vi "puff_stimulus_advanced.vi"(2 "Input Array":dbl[](array[numeric]), 3 "Cluster":T1) -> (0 "Timing array changed?":bool, 1 "Output Array":dbl[](array[numeric]))   [LabVIEW 2015]
panel:
  in  "Puff Stimulus Duration(ms)":i32[][](array[numeric]) min=4 max=65535
  in  "Fraction of time between is active":sgl[][](array[numeric]) min=5e-06 max=0.99995
  in  "stop":bool
  in  "OK Button":bool
  in  "Puff Stimulus Timing Array":dbl[](array[numeric])
  # "Duty Cycle"
  # "Switch time (ms)"
  # "Puff Stimulus Timing Array (ms)"
  # "Trigger signal duration (ms)"
  # "Switch time (ms)"
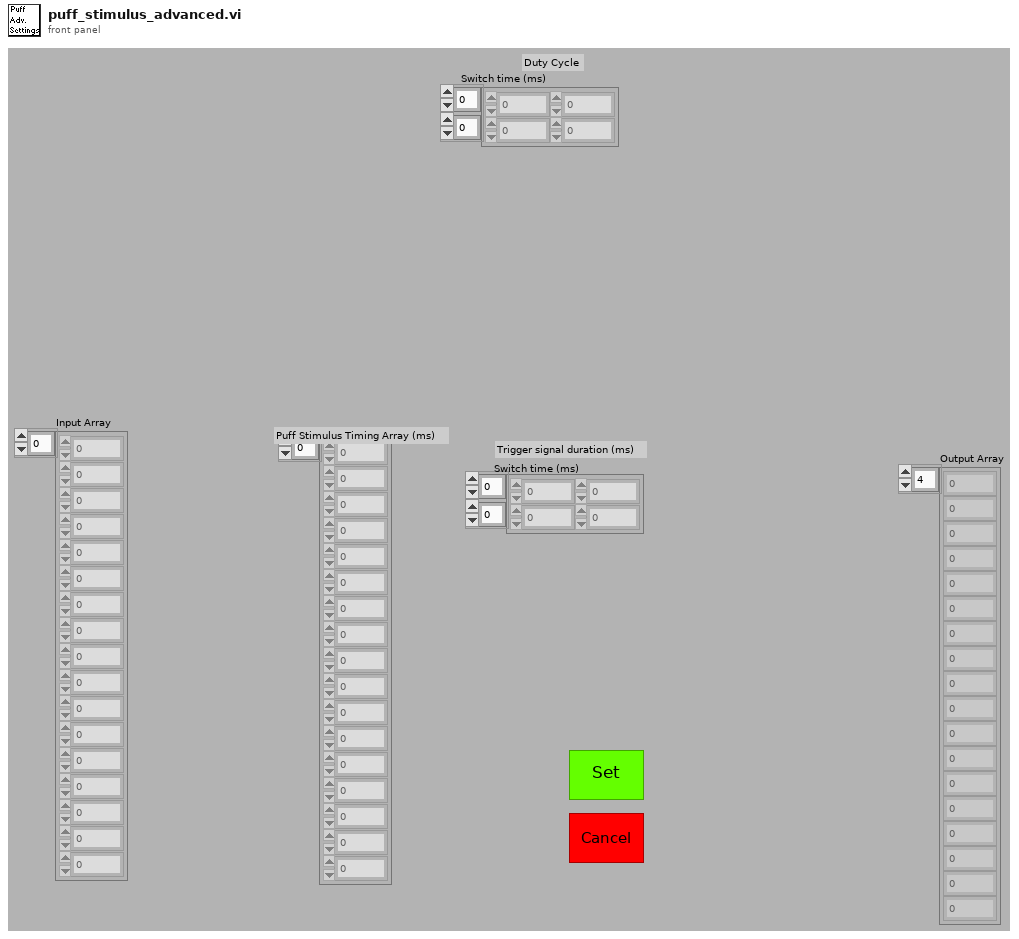
[diagram p1: front panel]
types:
  T1 = cluster{"puff fraction of time between is active":refnum<vi>, "time between puff onset":refnum<vi>}
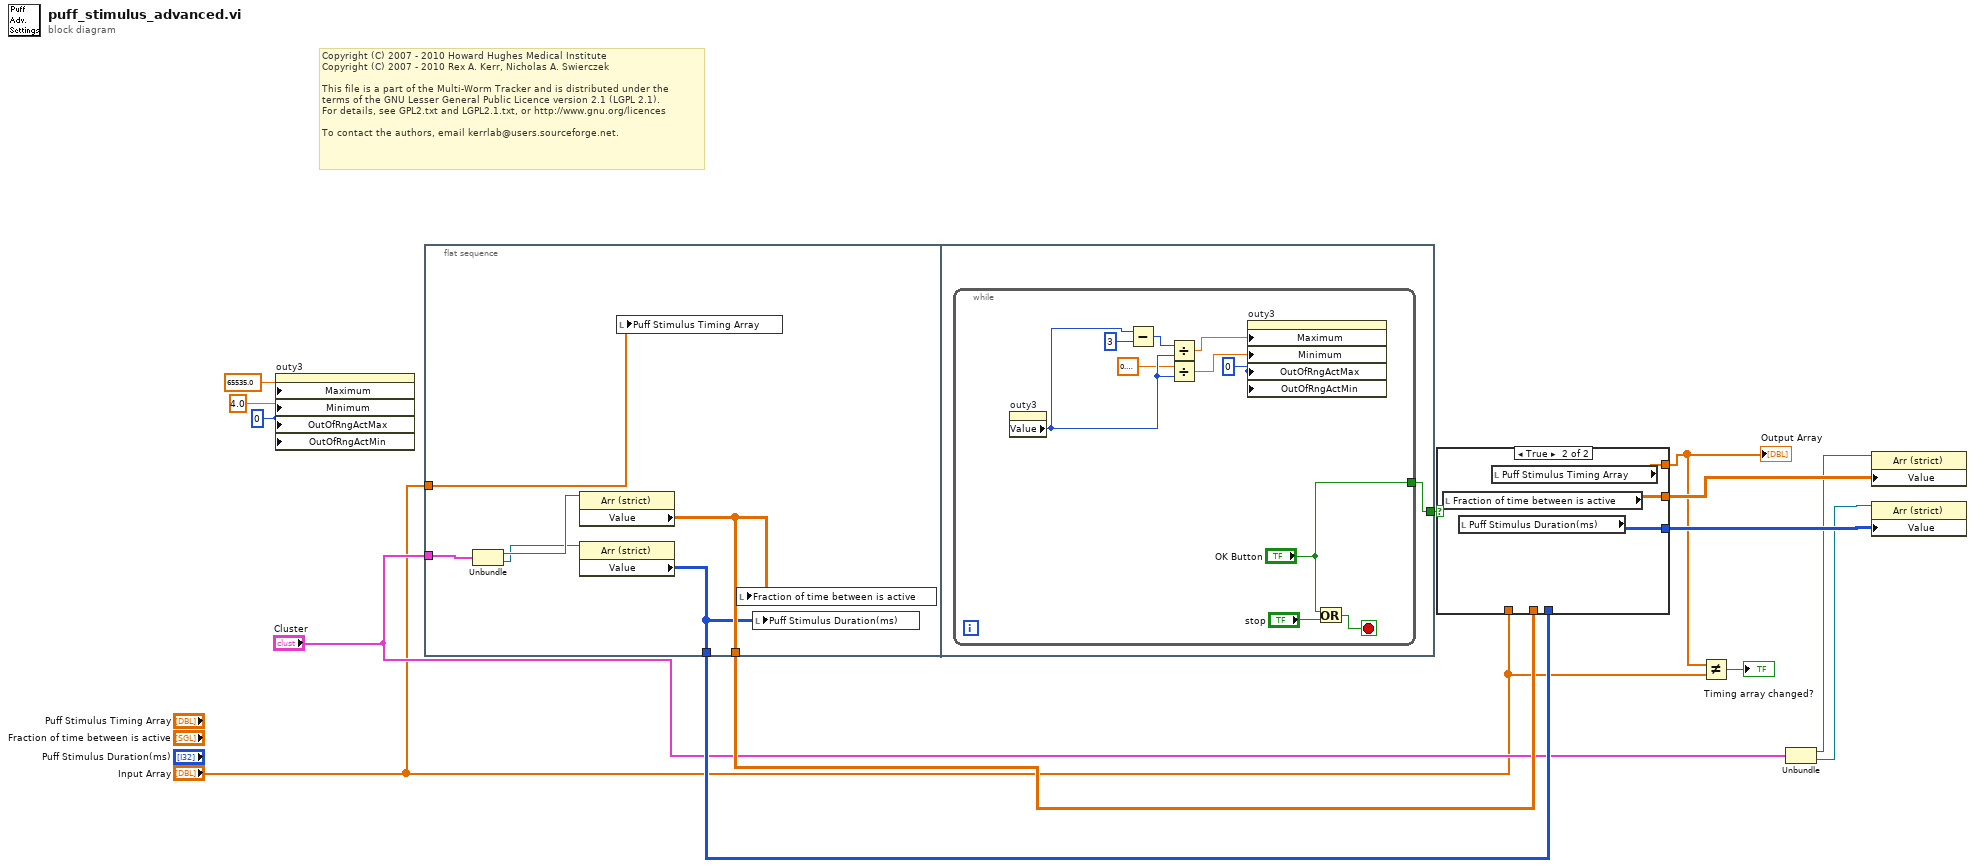
[diagram p0: block diagram]
diagram:
  w7 = u8 0 ("Response to Value Outside Limits:Maximum")
  # "Copyright (C) 2007 - 2010 Howard Hughes Medical Institute\nCopyright (C) 2007 - 2010 Rex A. Kerr, Nicholas A. Swierczek\n \nThis file is a part of the Multi-Worm Tracker and is distributed under the\nterms of the GNU Lesser General Public Licence version 2.1 (LGPL 2.1).\nFor details, see GPL2.txt and LGPL2.1.txt, or http://www.gnu.org/licences\n \nTo contact the authors, email kerrlab@users.sourceforge.net."
  n1 = property on="outy3" class="DigNum (strict)"("Maximum"=65535.0 ("x"), "Minimum"=4.0 ("Data Entry Limits:Minimum"), "OutOfRngActMax"=w7, "OutOfRngActMin"=w7) -> ()  [unwired: 2 in, 2 out]
  n2 = flat-sequence {
    tunnel: "Input Array" -> [w20]
    tunnel: "Cluster" -> [w19]
    tunnel: [w18] -> w6
    tunnel: [w17] -> w5
    tunnel: [w21] -> w14
    frame #0 {
      n3 = Unbundle(w19) -> ("puff fraction of time between is active"=w16:refnum<vi>, "time between puff onset"=w15:refnum<vi>)
      n4 = property class="Arr (strict)"(reference=w16) -> ("Value"=w18:sgl[][])  [unwired: 1 in, 2 out]
      n5 = property class="Arr (strict)"(reference=w15) -> ("Value"=w17:i32[][])  [unwired: 1 in, 2 out]
      n6 = local write "Puff Stimulus Timing Array"(w20) -> ()
      n7 = local write "Fraction of time between is active"(w18) -> ()
      n8 = local write "Puff Stimulus Duration(ms)"(w17) -> ()
    }
    frame #1 {
      n9 = while {
        tunnel: ["OK Button"] -> w21
        stop <- w31 stop-if-true
        w28 = u8 0 ("Response to Value Outside Limits:Maximum")
        n10 = property on="outy3" class="DigNum (strict)"() -> ("Value"=w27:i32)  [unwired: 2 in, 2 out]
        n11 = Subtract(x=w27, y=3) -> (x-y=w25:i32)
        n12 = Divide(x=w25, y=w27) -> (x/y=w26:dbl)
        n13 = Divide(x=sgl 0.3, y=w27) -> (x/y=w22:sgl)
        n14 = property on="outy3" class="DigNum (strict)"("Maximum"=w26, "Minimum"=w22, "OutOfRngActMax"=w28, "OutOfRngActMin"=w28) -> ()  [unwired: 2 in, 2 out]
        n15 = Or(x="OK Button", y="stop") -> (x .or. y?=w31:bool)
      }
    }
  }
  n16 = case shown="True" w14 {
    tunnel: "Input Array" -> [w34 _]
    tunnel: [w34 w37] -> w3
    tunnel: [w33 w36] -> w13
    tunnel: [w32 w35] -> w12
    tunnel: w6 -> [w33 _]
    tunnel: w5 -> [w32 _]
    frame False {
    }
    frame True {
      n17 = local read "Fraction of time between is active"() -> (w36:sgl[][])
      n18 = local read "Puff Stimulus Duration(ms)"() -> (w35:i32[][])
      n19 = local read "Puff Stimulus Timing Array"() -> (w37:dbl[])
    }
  }
  "Output Array" <- w3
  n20 = Not Equal?(x=w3, y="Input Array") -> (x != y?=→"Timing array changed?":bool)
  n21 = Unbundle("Cluster") -> ("puff fraction of time between is active"=w11:refnum<vi>, "time between puff onset"=w10:refnum<vi>)
  n22 = property class="Arr (strict)"(reference=w11, "Value"=w13) -> ()  [unwired: 1 in, 2 out]
  n23 = property class="Arr (strict)"(reference=w10, "Value"=w12) -> ()  [unwired: 1 in, 2 out]
